vi "como plasmar ecuaciones.vi"() -> ()   [LabVIEW 2021]
panel:
  out "Error":string
  out "x2":dbl
  out "x1":dbl
  in  "A":dbl
  in  "B":dbl
  in  "C":dbl
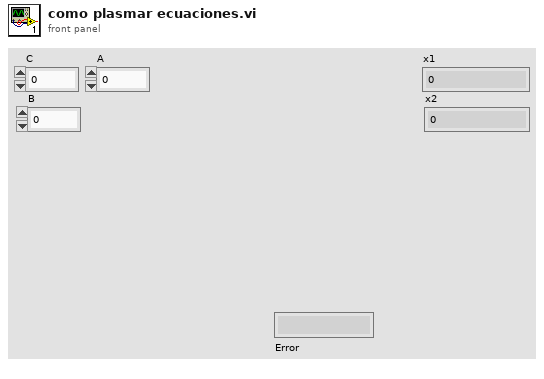
[diagram p1: front panel]
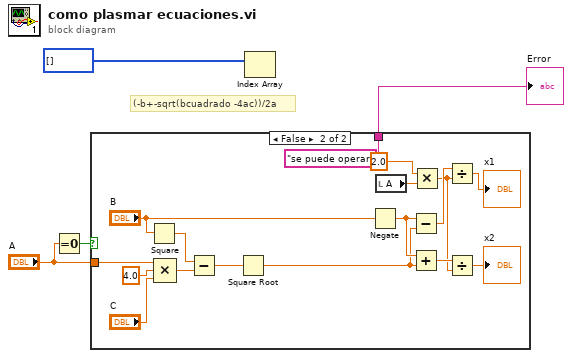
[diagram p0: block diagram]
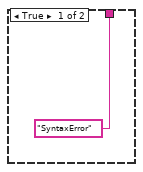
[diagram p2: hidden frame]
diagram:
  # "(-b+-sqrt(bcuadrado -4ac))/2a"
  n1 = Equal To 0?(x="A") -> (x = 0?=w2:bool)
  n2 = case shown="False" w2 {
    tunnel: "A" -> [_ w15]
    tunnel: ["SyntaxError" ("Error") "se puede operar" ("Error")] -> w1
    frame True {
    }
    frame False {
      n3 = Square(x="B") -> (x^2=w22:dbl)
      n4 = Compound Arithmetic op=MULTIPLY(w15, 4.0 ("value"), "C") -> (w9:dbl)
      n5 = Subtract(x=w22, y=w9) -> (x-y=w21:dbl)
      n6 = Square Root(x=w21) -> (sqrt(x)=w7:dbl)
      n7 = Negate(x="B") -> (-x=w8:dbl)
      n8 = local read "A"() -> (w12:dbl)
      n9 = Subtract(x=w8, y=w7) -> (x-y=w19:dbl)
      n10 = Add(x=w8, y=w7) -> (x+y=w18:dbl)
      n11 = Multiply(x=2.0, y=w12) -> (x*y=w10:dbl)
      n12 = Divide(x=w19, y=w10) -> (x/y=→"x1":dbl)
      n13 = Divide(x=w18, y=w10) -> (x/y=→"x2":dbl)
    }
  }
  "Error" <- w1
  n14 = Index Array(array=i32[] []) -> ()  [unwired: 1 in, 1 out]
